vi "FPGA_EncoderOpen WO Configuration.vi"(8 "DeviceStatus":errorcluster, 11 "EncoderIndex":T1) -> (0 "error out":errorcluster, 3 "Encoder Reference":T2)   [LabVIEW 2017]
uses:
  <vilib>/Rock Robotics/SystemInterfaces/Encoder/FPGA_EncoderDevRef.ctl
  <vilib>/Rock Robotics/SystemInterfaces/Encoder/FPGA_EncoderIdx.ctl
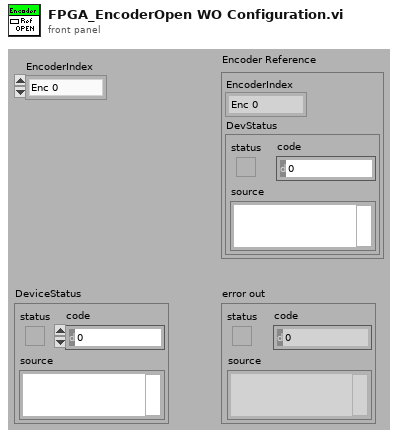
[diagram p1: front panel]
types:
  T1 = typedef "FPGA_EncoderIdx.ctl" = enum8{"Enc 0", "Enc 1", "Enc 2", "Enc 3", "Enc 4", "Enc 5", "Enc 6", "Enc 7", "Invalid"}
  T2 = typedef "FPGA_EncoderDevRef.ctl" = cluster{"EncoderIndex":T1, "DevStatus":errorcluster}
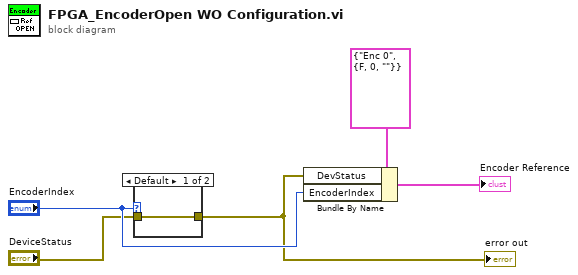
[diagram p0: block diagram]
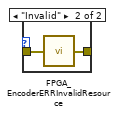
[diagram p2: hidden frame]
diagram:
  n1 = case shown="Default" "EncoderIndex" {
    tunnel: [w6 w8] -> w2
    tunnel: "DeviceStatus" -> [w6 w7]
    frame Default {
    }
    frame "Invalid" {
      n2 = call <vilib>:"FPGA_EncoderERRInvalidResource.vi"("error in (no error)"=w7) -> ("error out"=w8:errorcluster)
    }
  }
  "error out" <- w2
  n3 = Bundle By Name(cluster=T2 {"EncoderIndex"=enum."Enc 0", "DevStatus"={"status"=FALSE, "code"=0, "source"=""}} ("Encoder Reference out"), "DevStatus"=w2, "EncoderIndex"="EncoderIndex") -> (→"Encoder Reference":T2)
